vi "Create File.vi"(8 "error in":errorcluster, 11 "TDMS in":refnum<class "TDMS.lvclass">) -> (0 "error out":errorcluster, 3 "TDMS out":refnum<class "TDMS.lvclass">)   [LabVIEW 2019, in "TDMS.lvlib" / "TDMS.lvclass"]
uses:
  TDMS.lvclass
  C:/Users/Public/Documents/Development/builds/Tools/Report.lvlibp/Report.lvclass
  TDMS.lvclass/TDMS.ctl
  Accessors/Write TDMS Ref.vi
  builds/Tools/Report.lvlibp/Accessors/Read Report Path.vi
  builds/Tools/Report.lvlibp/Accessors/Read Test Name.vi
  builds/Tools/Report.lvlibp/Accessors/Read UUT_Name.vi
  builds/Tools/Report.lvlibp/Accessors/Read Test Date.vi
  builds/Tools/Report.lvlibp/Accessors/Read Test Time.vi
  builds/Tools/Report.lvlibp/Accessors/Write Report Path.vi
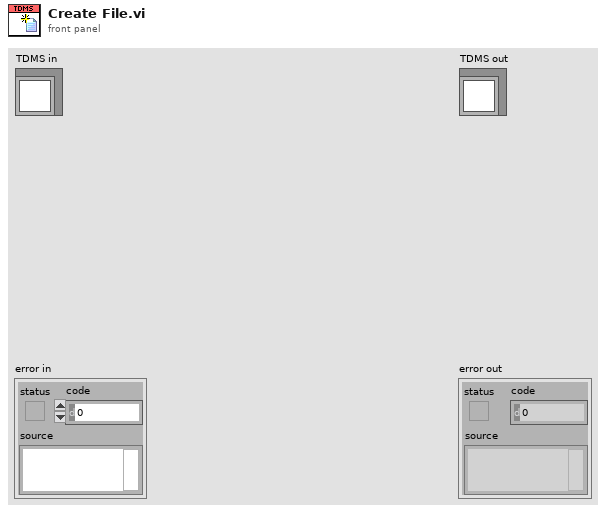
[diagram p1: front panel]
types:
  T1 = enum16{"open", "open or create", "create or replace", "create", "open (read-only)"}
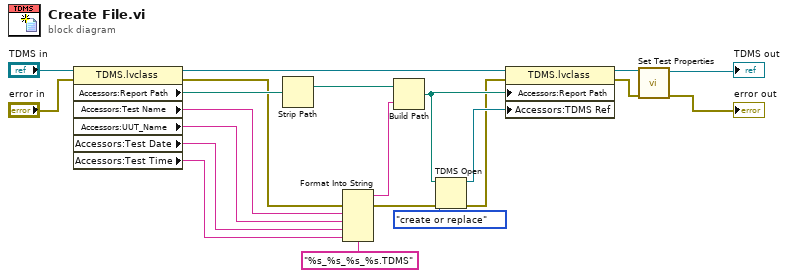
[diagram p0: block diagram]
diagram:
  n1 = property class="TDMS.lvclass"(reference="TDMS in", error in="error in") -> (reference out=w18:refnum<class "TDMS.lvclass">, error out=w8:errorcluster, "Accessors:Report Path"=w19:path, "Accessors:Test Name"=w4:string, "Accessors:UUT_Name"=w3:string, "Accessors:Test Date"=w2:string, "Accessors:Test Time"=w1:string)
  n2 = Strip Path(path=w19) -> (stripped path=w16:path)  [unwired: 1 out]
  n3 = Format Into String(format string="%s_%s_%s_%s.TDMS", error in=w8, w4, w3, w2, w1) -> (resulting string=w5:string, error out=w7:errorcluster)  [unwired: 1 in]
  n4 = Build Path(base path=w16, name or relative path=w5) -> (appended path=w17:path)
  n5 = TDMS Open(8:w7, 10:T1."create or replace" ("operation (0:open)"), 11:w17) -> (0:w13:errorcluster, 3:w15:refnum<k34>)  [unwired: 4 in]
  n6 = property class="TDMS.lvclass"(reference=w18, error in=w13, "Accessors:Report Path"=w17, "Accessors:TDMS Ref"=w15) -> (reference out=w12:refnum<class "TDMS.lvclass">, error out=w11:errorcluster)
  n7 = call "Set Test Properties.vi"("error in"=w11, "TDMS in"=w12) -> ("error out"=→"error out":errorcluster, "TDMS out"=→"TDMS out":refnum<class "TDMS.lvclass">)  [unwired: 8 in]
